vi "Test Insert Tables without data.vi"(11 "Test Case In":refnum<class "Test Open Xml.lvclass">) -> (0 "error out":errorcluster, 3 "Test Case Out":refnum<class "Test Open Xml.lvclass">)   [LabVIEW 2020, in "Test Open Xml.lvclass"]
uses:
  Test Open Xml.lvclass
  Source/Open Xml.lvlib
  0a0d70f3-36fe-46ba-8b3e-e6c07e708d9f.vi
panel:
  out "Sheet Name":string
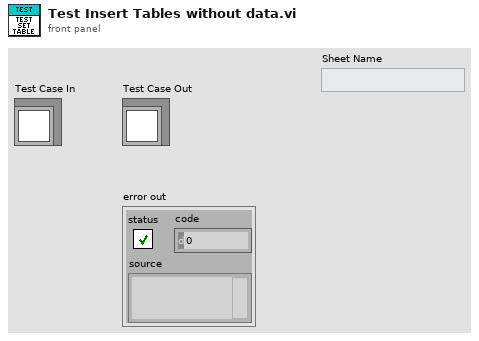
[diagram p1: front panel]
types:
  T1 = cluster{"Sheet Name":string, "Name":string, "Display Name":string, "Range or Cell Address":string}
  T2 = cluster{"Sheet Name":string, "Name":string, "Display Name":string, "Range":string}
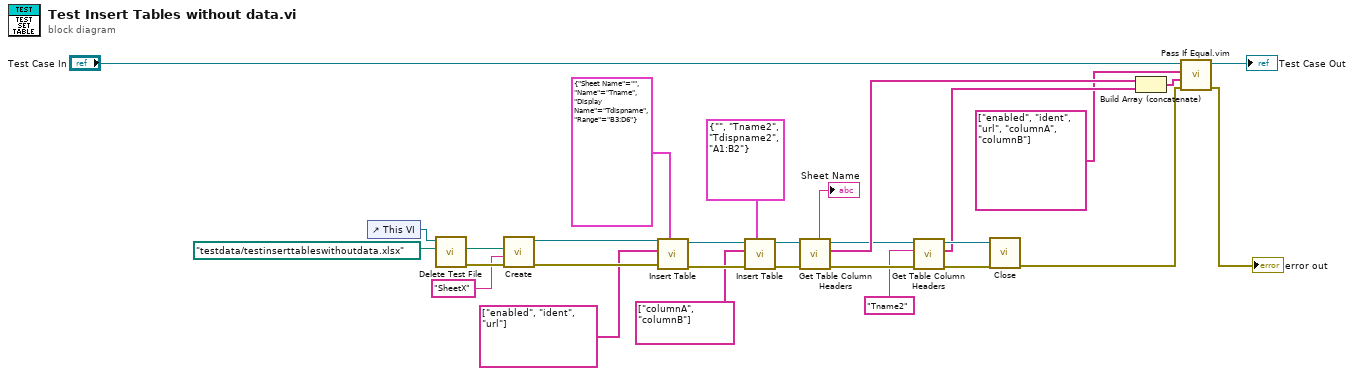
[diagram p0: block diagram]
diagram:
  n1 = control-ref of="This VI"() -> (w19:refnum<vi>)
  n2 = call "Delete Test File.vi"("name or relative path"=path "testdata/testinserttableswithoutdata.xlsx", "VI in"=w19) -> ("error out"=w20:errorcluster, "deleted path"=w21:path)  [unwired: 8 in]
  n3 = call "Create.vi"("error in"=w20, "SheetName"="SheetX", "Path"=w21) -> ("error out"=w16:errorcluster, "SpreadsheetDoc"=w17:refnum<k24>)  [unwired: 7 in]
  n4 = call "Insert Table.vi"("Location"=T2 {"Sheet Name"="", "Name"="Tname", "Display Name"="Tdispname", "Range"="B3:D6"}, "error in"=w16, "Header Names"=string[] ["enabled", "ident", "url"], "SpreadsheetDoc in"=w17) -> ("error out"=w23:errorcluster, "SpreadsheetDoc out"=w11:refnum<k24>)  [unwired: 6 in]
  n5 = call "Insert Table.vi"("Location"=T1 {"Sheet Name"="", "Name"="Tname2", "Display Name"="Tdispname2", "Range or Cell Address"="A1:B2"}, "error in"=w23, "Header Names"=string[] ["columnA", "columnB"], "SpreadsheetDoc in"=w11) -> ("error out"=w12:errorcluster, "SpreadsheetDoc out"=w10:refnum<k24>)  [unwired: 6 in]
  n6 = call "Get Table Column Headers.vi"("error in"=w12, "SpreadsheetDoc in"=w10) -> ("error out"=w25:errorcluster, "Headers"=w24:string[], "SpreadsheetDoc out"=w6:refnum<k24>, "Sheet Name out"=→"Sheet Name":string)  [unwired: 6 in]
  n7 = call "Get Table Column Headers.vi"("error in"=w25, "Table Name"="Tname2", "SpreadsheetDoc in"=w6) -> ("error out"=w7:errorcluster, "Headers"=w3:string[], "SpreadsheetDoc out"=w5:refnum<k24>)  [unwired: 5 in, 1 out]
  n8 = call "Close.vi"("error in"=w7, "SpreadsheetDoc"=w5) -> ("error out"=w26:errorcluster)  [unwired: 9 in]
  n9 = Build Array (concatenate)(w24, w3) -> (w4:string[])
  n10 = call "Pass If Equal.vim"("error in (no error)"=w26, "Actual"=w4, "Expected"=string[] ["enabled", "ident", "url", "columnA", "columnB"] ("Headers"), "LUnit Test Case In"="Test Case In") -> ("error out"=→"error out":errorcluster, "LUnit Test Case Out"=→"Test Case Out":refnum<class "Test Open Xml.lvclass">)  [unwired: 6 in]
